vi "WriteResults_Manual.vi"(7 "Timestamp":string, 8 "error in":errorcluster, 9 "Result":string, 10 "Commands":string, 11 "refnum in":refnum<file>) -> (0 "error out":errorcluster, 3 "refnum out":refnum<file>)   [LabVIEW 2018]
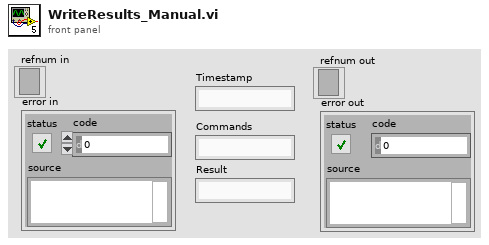
[diagram p1: front panel]
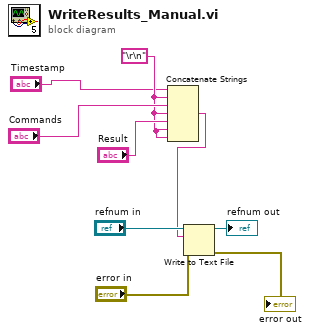
[diagram p0: block diagram]
diagram:
  w2 = "\r\n"
  n1 = Concatenate Strings("Timestamp", w2, "Commands", w2, "Result", w2, w2) -> (w3:string)
  n2 = Write to Text File(file (use dialog)="refnum in", text=w3, error in="error in") -> (refnum out=→"refnum out":refnum<file>, error out=→"error out":errorcluster)  [unwired: 1 in, 1 out]
